vi "Paths Write 2.vi"(4 "error in (no error)":errorcluster, 5 "Value":T3={"Webview2 Native"=path "C:/Users/kleins/Desktop/webview2/microsoft.web.webview2.1.0.1370.28/build/native", "Edge Application"=path "", "User Data"=path ""}, 6 "Container State":T2, 7 "Display State In":T1) -> (0 "error out":errorcluster, 3 "Display State Out":T1)   [LabVIEW 2020, in "WebView2 Control.xctl"]
uses:
  WebView2 Control.xctl
  <vilib>/_xctls/Container State.ctl
  Webview2 Lib/WebView2 Control Object/Paths.ctl
  State.ctl
  Webview2 Lib/WebView2 Control Object/WebView2 Control.lvclass
  <vilib>/_xctls/XControlSupport.lvlib
panel:
  # "Replace the Value Control below with a Control of desired type.\nDo not remove this Control or the others from the connector pane.\nDo not change the connector pane pattern.\nThe Value control should always be the third terminal from top on the input side in the connector pane."
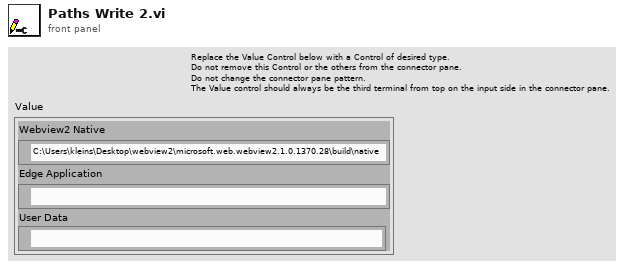
[diagram p1: front panel]
types:
  T1 = typedef "WebView2 Control.xctl/State.ctl" = cluster{"Control Object Ref":refnum<data-value>}
  T2 = typedef "XControlSupport.lvlib/Container State.ctl" = cluster{"Indicator?":bool, "Run Mode?":bool, " Refnum":refnum<vi>}
  T3 = typedef "WebView2.lvlib/WebView2 Control.lvclass/Paths.ctl" = cluster{"Webview2 Native":path, "Edge Application":path, "User Data":path}
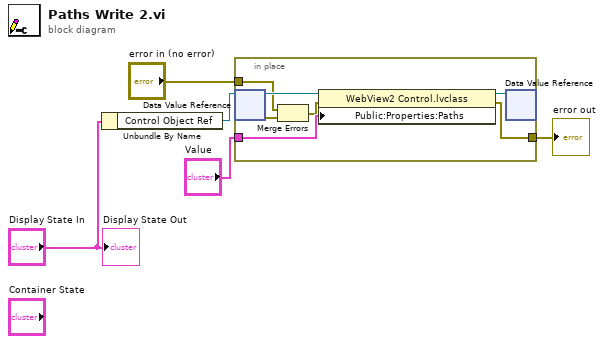
[diagram p0: block diagram]
diagram:
  n1 = Unbundle By Name("Display State In") -> ("Control Object Ref"=w4:refnum<data-value>)
  n2 = in-place {
    in-place-border: "Value" -> [w10]
    in-place-border: [w8] -> w2
    in-place-border: "error in (no error)" -> [w6]
    n3 = in-place-dvr #1(w4) -> (w12:refnum<class "WebView2 Control.lvclass">, w9:errorcluster)
    n4 = Merge Errors(w6, w9) -> (w7:errorcluster)
    n5 = property class="WebView2 Control.lvclass"(reference=w12, error in=w7, "Public:Properties:Paths"=w10) -> (reference out=w11:refnum<class "WebView2 Control.lvclass">, error out=w8:errorcluster)
    n6 = in-place-dvr #1(w11) -> ()  [unwired: 2 out]
  }
  "error out" <- w2
  "Display State Out" <- "Display State In"
